vi "Align Mask and Signal - wfm.vi"(0 "Waveform":waveform(dbl)={"t0"=timestamp(0 s since 1904-01-01), "dt"=0.0, "Y"=[]}, 5 "trigger index":i32, 7 "upper limit":waveform(dbl), 9 "lower limit":waveform(dbl), 11 "error in (no error)":errorcluster, 12 "Mask Selector":u16(ring) items=["ITU", "EIA/TIA 547-1989"]) -> (3 "Subset Waveform":waveform(dbl), 4 "Waveform out":waveform(dbl), 6 "upper limit out":waveform(dbl), 8 "lower limit out":waveform(dbl), 15 "error out":errorcluster)   [LabVIEW 2013]
uses:
  <vilib>/Waveform/WDTOps.llb/WDT Number of Waveform Samples DBL.vi
  <vilib>/Waveform/WDTOps.llb/WDT Get Waveform Subset DBL (LV80).vi
  <vilib>/Waveform/WDTOps.llb/WDT Align Waveform Timestamps DBL.vi
  <vilib>/Analysis/NI_AALBase.lvlib
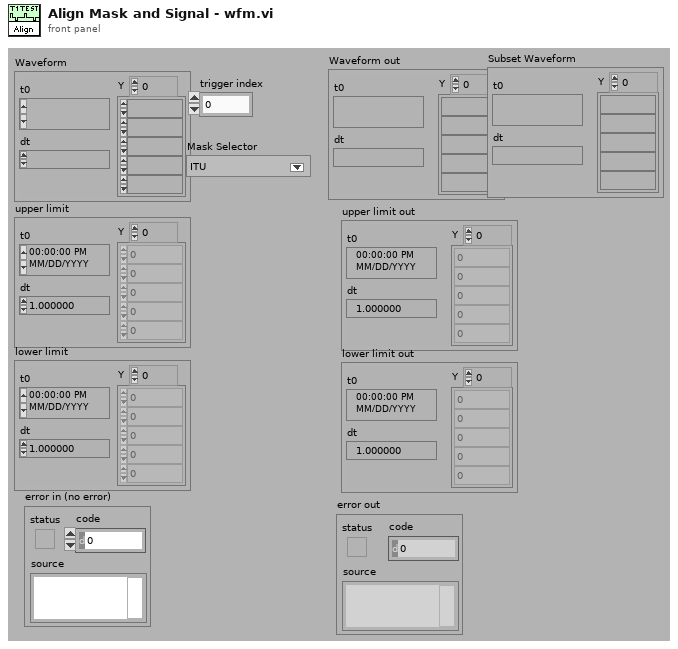
[diagram p1: front panel]
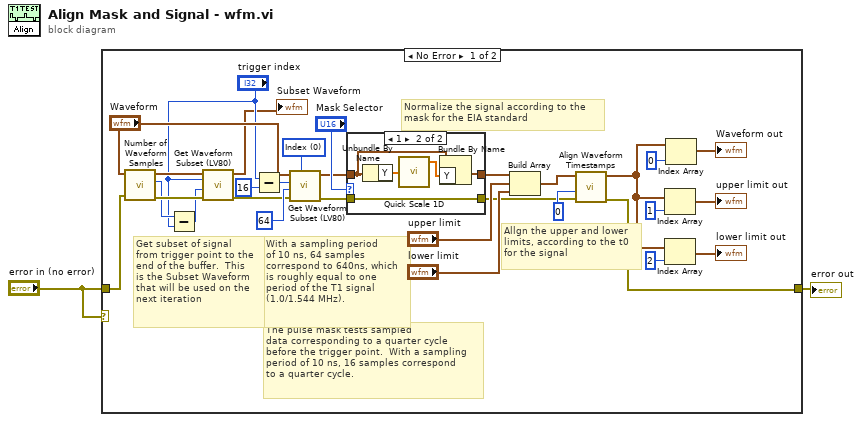
[diagram p0: block diagram]
diagram:
  n1 = case shown="No Error" "error in (no error)" {
    tunnel: "error in (no error)" -> [w15 w40]
    tunnel: [w21 w40] -> w1
    frame No Error {
      w16 = u16 0 items=["Index", "Relative Time"] ("Mode")
      # "Normalize the signal according to the \nmask for the EIA standard"
      # "Allgn the upper and lower\nlimits, according to the t0 \nfor the signal"
      # "The pulse mask tests sampled\ndata corresponding to a quarter cycle\nbefore the trigger point.  With a sampling\nperiod of 10 ns, 16 samples correspond\nto a quarter cycle."
      # "With a sampling period\nof 10 ns, 64 samples\ncorrespond to 640ns, which\nis roughly equal to one\nperiod of the T1 signal\n(1.0/1.544 MHz)."
      # "Get subset of signal\nfrom trigger point to the\nend of the buffer.  This\nis the Subset Waveform\nthat will be used on the \nnext iteration"
      n2 = call-poly <vilib>:"Number of Waveform Samples.vi"("error in (no error)"=w15, "waveform in"="Waveform") -> ("error out"=w13:errorcluster, "number of samples"=w11:i32, "waveform out"=w14:waveform(dbl))  [unwired: 7 in]
      n3 = Subtract(x=w11, y="trigger index") -> (x-y=w9:i32)
      n4 = call-poly <vilib>:"Get Waveform Subset (LV80).vi"("error in (no error)"=w13, "duration"=w9, "start samples/time"="trigger index", "waveform in"=w14) -> ("error out"=w12:errorcluster, "waveform out"=→"Subset Waveform":waveform(dbl))  [unwired: 2 in, 2 out]
      n5 = Subtract(x="trigger index", y=16) -> (x-y=w19:i32)
      n6 = call-poly <vilib>:"Get Waveform Subset (LV80).vi"("start/duration format"=w16, "error in (no error)"=w12, "duration"=64 ("Array Length"), "start samples/time"=w19, "waveform in"="Waveform") -> ("error out"=w6:errorcluster, "waveform out"=w4:waveform(dbl))  [unwired: 1 in, 2 out]
      n7 = case shown="1" "Mask Selector" {
        tunnel: w6 -> [w34 w39]
        tunnel: [w34 w39] -> w5
        tunnel: w4 -> [w33 w37]
        tunnel: [w33 w35] -> w3
        frame 0, Default {
        }
        frame 1 {
          n8 = Unbundle By Name(w37) -> ("Y"=w38:dbl[])
          n9 = call <vilib>:"Quick Scale 1D.vi"("X"=w38) -> ("Y[i]=X[i]/Max|X|"=w36:dbl[])  [unwired: 2 out]
          n10 = Bundle By Name(cluster=w37, "Y"=w36) -> (w35:waveform(dbl))
        }
      }
      n11 = Build Array(w3, "upper limit", "lower limit") -> (w30:waveform(dbl)[])
      n12 = call-poly <vilib>:"Align Waveform Timestamps.vi"("error in (no error)"=w5, "index"=0 ("Index"), "waveforms in"=w30) -> ("error out"=w21:errorcluster, "waveforms out"=w28:waveform(dbl)[])  [unwired: 7 in]
      n13 = Index Array(array=w28, index=1 ("Index")) -> (element=→"upper limit out":waveform(dbl))
      n14 = Index Array(array=w28, index=2 ("Index")) -> (element=→"lower limit out":waveform(dbl))
      n15 = Index Array(array=w28, index=0 ("Index")) -> (element=→"Waveform out":waveform(dbl))
    }
    frame Error {
    }
  }
  "error out" <- w1
